vi "Excel - ActiveX Event Callback.vi"() -> ()   [LabVIEW 2023]
doc: "This example uses the Microsoft Excel Application ActiveX automation refnum. It demonstrates how to register an ActiveX event callback and extract event data."
panel:
  in  "Stop":bool
  # "Overview: Demonstrates how to configure an ActiveX Event Callback, and modify the ActiveX object when the callback VI executes.\nRequirements: Windows with Microsoft Excel\nInstructions:\n1. Run the VI.\n2. After Microsoft Excel opens, create a new workbook by selecting File > New > Blank Workbook.\n3. Observe that the new workbook is populated with data specified by the callback VI.\n4. Click Stop to stop the VI."
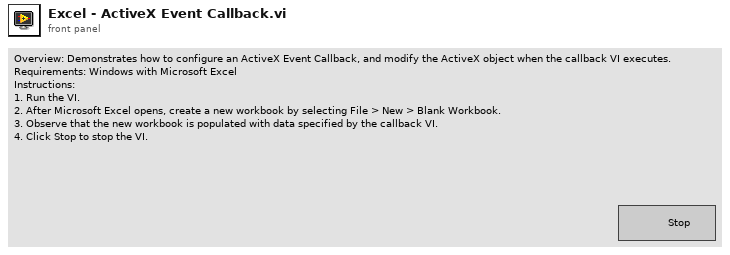
[diagram p1: front panel]
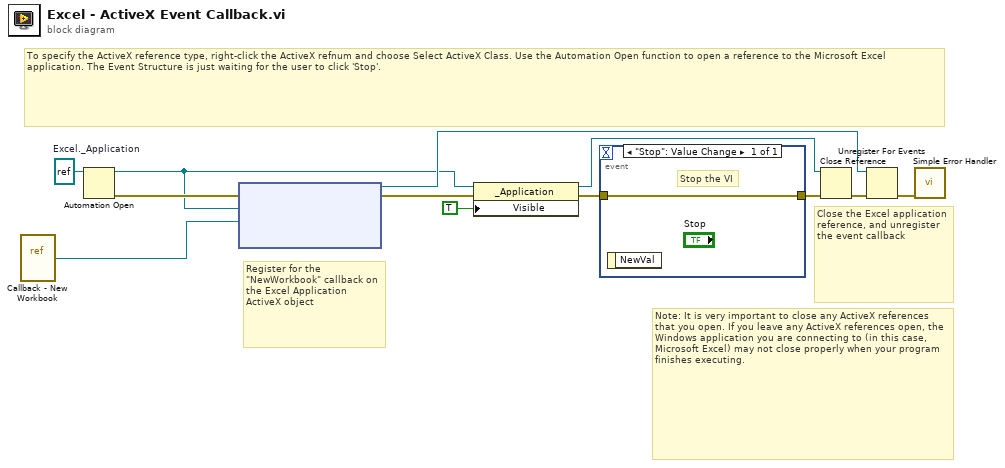
[diagram p0: block diagram]
diagram:
  w8 = refnum<k7> refnum  # Excel._Application
  # "Note: It is very important to close any ActiveX references that you open. If you leave any ActiveX references open, the Windows application you are connecting to (in this case, Microsoft Excel) may not close properly when your program finishes executing."
  # "To specify the ActiveX reference type, right-click the ActiveX refnum and choose Select ActiveX Class. Use the Automation Open function to open a reference to the Microsoft Excel application. The Event Structure is just waiting for the user to click 'Stop'."
  # "Close the Excel application reference, and unregister the event callback"
  # "Register for the \"NewWorkbook\" callback on the Excel Application ActiveX object"
  n1 = vi-ref "Callback - New Workbook.vi"() -> ("vi reference"=w12:refnum<vi>)
  n2 = Automation Open(Automation Refnum=w8) -> (Automation Refnum=w4:refnum<k7>, error out=w7:errorcluster)  [unwired: 3 in]
  n3 = node(w7, w4, w12) -> (w9:refnum<k27>, w5:errorcluster)  [unwired: 2 in]
  n4 = property class="_Application"(reference=w4, error in=w5, "Visible"=TRUE) -> (reference out=w1:refnum<k7>, error out=w3:errorcluster)
  n5 = event shown="[0] \"Stop\": Value Change" {
    selector: _ -> [_]
    dyn-events: _ -> [_]
    timeout: _ -> [_]
    tunnel: w3 -> [w13]
    tunnel: [w13] -> w11
    event "Stop": Value Change {
      # "Stop the VI"
      n6 = event-data() -> ()  [unwired: 1 in, 1 out]
    }
  }
  n7 = Close Reference(reference=w1, error in (no error)=w11) -> (error out=w6:errorcluster)
  n8 = Unregister For Events(event registration refnum=w9, error in=w6) -> (error out=w10:errorcluster)
  n9 = call <vilib>:"Simple Error Handler.vi"("error in (no error)"=w10) -> ()  [unwired: 4 in, 5 out]
